vi "Player Info.vi"(11 "Hesitant Wolf in":refnum<class "Hesitant Wolf.lvclass">) -> (1 "Victory Speech":string, 2 "Name":string, 3 "Hesitant Wolf out":refnum<class "Hesitant Wolf.lvclass">)   [LabVIEW 2015, in "Hesitant Wolf.lvclass"]
uses:
  Hesitant Wolf.lvclass
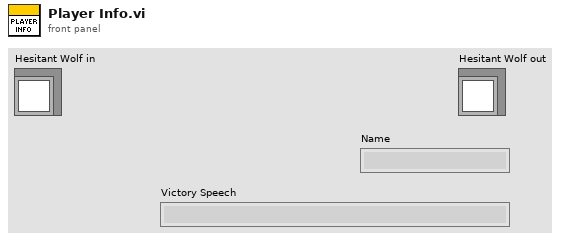
[diagram p1: front panel]
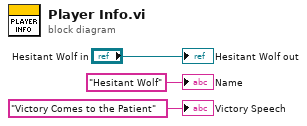
[diagram p0: block diagram]
diagram:
  "Hesitant Wolf out" <- "Hesitant Wolf in"
  "Name" <- "Hesitant Wolf" ("Name")
  "Victory Speech" <- "Victory Comes to the Patient" ("Victory Speech")
